vi "Iteration Status Update.vi"(6 "Output Closed?":bool, 11 "Worker Block In":T1={"Block Status"=refnum, "Command Queue"=refnum, "Status"={"Block Status"={"State"=enum."Init", "Next State"=enum."Idle", "Runs"=0, "i"=0, "Init"=FALSE, "Started"=FALSE, "Closing"=FALSE, "Step"=FALSE, "Phase"=enum."N/A", "Worker"=""}, "Error"={"status"=FALSE, "code"=0, "source"=""}}}) -> (3 "Worker Block":T1={"Block Status"=refnum, "Command Queue"=refnum, "Status"={"Block Status"={"State"=enum."Init", "Next State"=enum."Idle", "Runs"=0, "i"=0, "Init"=FALSE, "Started"=FALSE, "Closing"=FALSE, "Step"=FALSE, "Phase"=enum."N/A", "Worker"=""}, "Error"={"status"=FALSE, "code"=0, "source"=""}}}, 5 "Stop Block":bool)   [LabVIEW 2022 SP3, in "FlexBlocks Support.lvlib"]
uses:
  FlexBlocks Support.lvlib
  Worker Block.ctl
  Block Status with Error.ctl
  Block Status.ctl
  Block State.ctl
  Block Phase.ctl
  Block Command.ctl
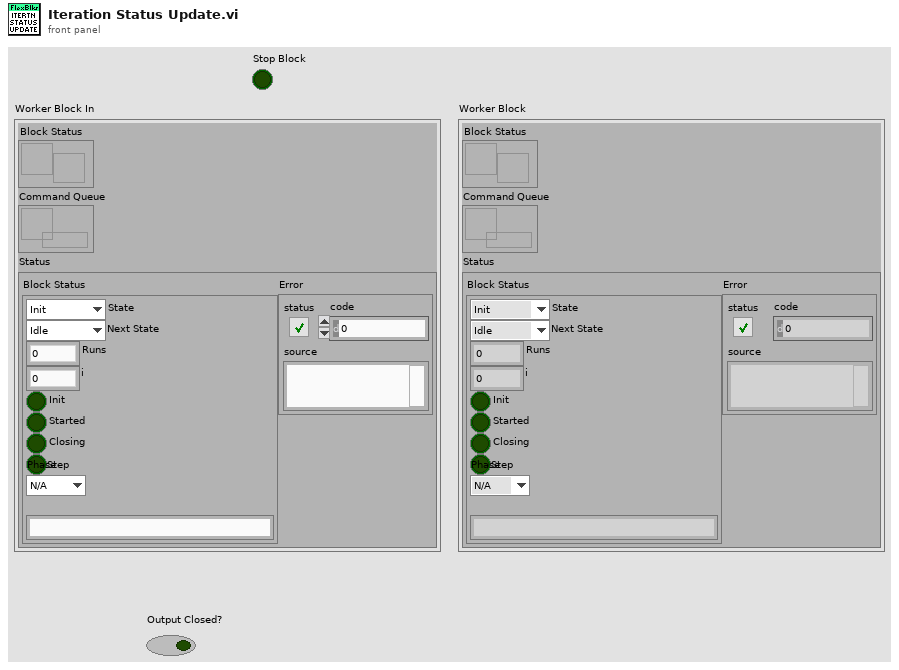
[diagram p1: front panel]
types:
  T1 = typedef "FlexBlocks Support.lvlib/Worker Block.ctl" = cluster{"Block Status":refnum<user-event>, "Command Queue":refnum<queue>, "Status":T2}
  T2 = typedef "FlexBlocks Support.lvlib/Block Status with Error.ctl" = cluster{"Block Status":T3, "Error":errorcluster}
  T3 = typedef "FlexBlocks Support.lvlib/Block Status.ctl" = cluster{"State":T4, "Next State":T4, "Runs":u32, "i":i32, "Init":bool, "Started":bool, "Closing":bool, "Step":bool, "Phase":T5, "Worker":string}
  T4 = typedef "FlexBlocks Support.lvlib/Block State.ctl" = enum16{"Idle", "Init", "Start", "Run", "Stop", "Close"}
  T5 = typedef "FlexBlocks Support.lvlib/Block Phase.ctl" = enum16{"N/A", "Read", "Work", "Write"}
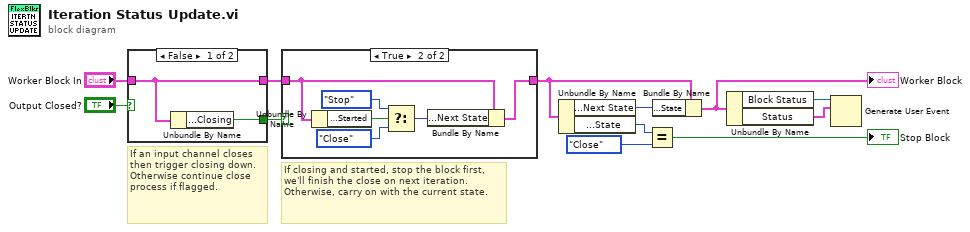
[diagram p0: block diagram]
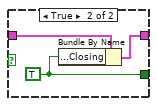
[diagram p3: hidden frame]
diagram:
  # "If closing and started, stop the block first, we'll finish the close on next iteration. Otherwise, carry on with the current state."
  # "If an input channel closes then trigger closing down. Otherwise continue close process if flagged."
  n1 = case shown="False" "Output Closed?" {
    tunnel: "Worker Block In" -> [w14 w17]
    tunnel: [w14 w16] -> w11
    tunnel: [w13 w15] -> w10
    frame False {
      n2 = Unbundle By Name(w14) -> ("Status.Block Status.Closing"=w13:bool)
    }
    frame True {
      w15 = TRUE ("Status.Block Status.Closing")
      n3 = Bundle By Name(cluster=w17, "Status.Block Status.Closing"=w15) -> (w16:T1)
    }
  }
  n4 = case shown="True" w10 {
    tunnel: w11 -> [w18 w21]
    tunnel: [w18 w19] -> w5
    frame False {
    }
    frame True {
      n5 = Unbundle By Name(w21) -> ("Status.Block Status.Started"=w23:bool)
      n6 = Select(t=Block_State."Stop" ("Block State"), s=w23, f=Block_State."Close" ("Block State")) -> (s? t:f=w20:T4)
      n7 = Bundle By Name(cluster=w21, "Status.Block Status.Next State"=w20) -> (w19:T1)
    }
  }
  n8 = Unbundle By Name(w5) -> ("Status.Block Status.Next State"=w4:T4, "Status.Block Status.State"=w8:T4)
  n9 = Equal?(x=w8, y=Block_State."Close") -> (x = y?=→"Stop Block":bool)
  n10 = Bundle By Name(cluster=w5, "Status.Block Status.State"=w4) -> (w3:T1)
  "Worker Block" <- w3
  n11 = Unbundle By Name(w3) -> ("Block Status"=w2:refnum<user-event>, "Status"=w1:T2)
  n12 = Generate User Event(user event=w2, event data cluster=w1) -> ()  [unwired: 2 in, 2 out]
